vi "HTTP Client Abstract Tree.vi"() -> ()   [LabVIEW 2021]
uses:
  Classes/HTTP Client Base/HTTP Client Base.lvclass
  C:/Users/bjustice/Documents/GitHub/HTTP-Client-Abstract/lv_src/Classes/HTTP Client Abstract/HTTP Client Abstract.lvclass
  Classes/HTTP Client reqwest/HTTP Client reqwest.lvclass
  Classes/HTTP Client Advanced/HTTP Client Advanced.lvclass
  Classes/HTTP Client Abstract/HTTP Client Abstract.lvclass
panel:
  out "Array":string[][](array[string])
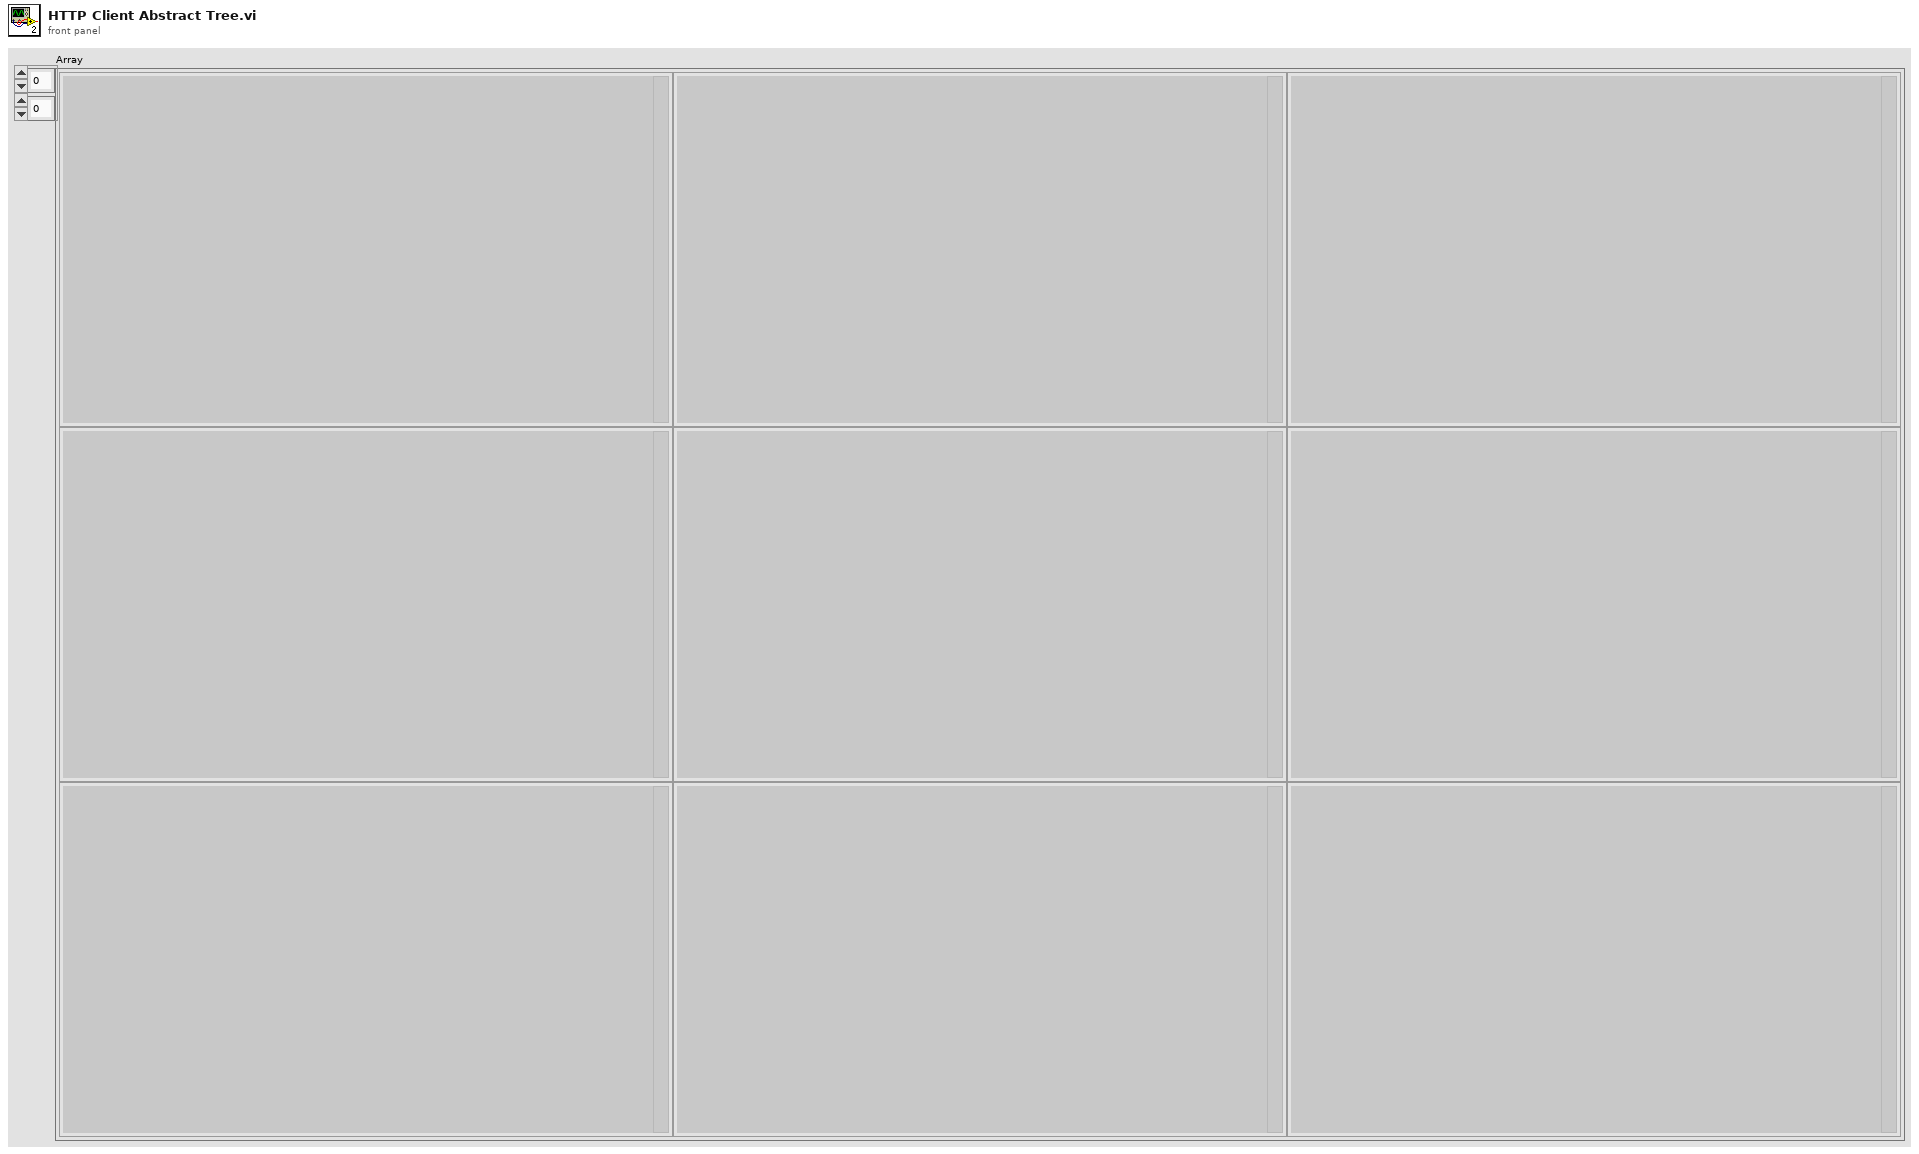
[diagram p1: front panel]
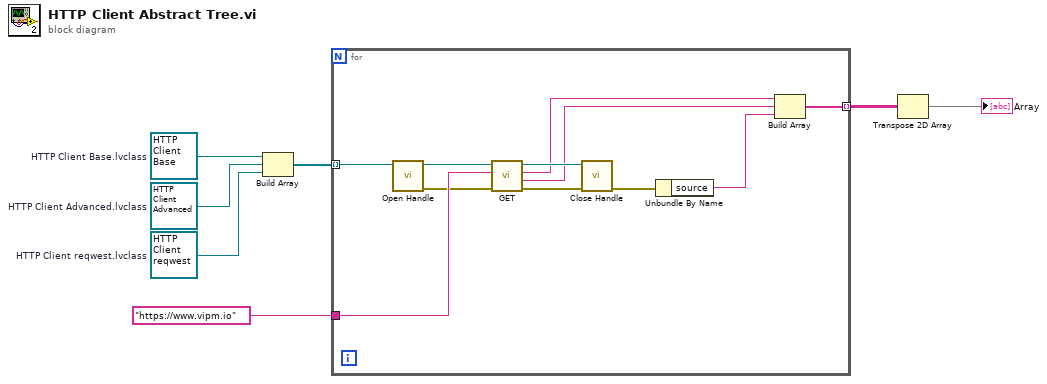
[diagram p0: block diagram]
diagram:
  w7 = refnum<class "HTTP Client Advanced.lvclass"> refnum  # HTTP Client Advanced.lvclass
  w5 = refnum<class "HTTP Client reqwest.lvclass"> refnum  # HTTP Client reqwest.lvclass
  w6 = refnum<class "HTTP Client Base.lvclass"> refnum  # HTTP Client Base.lvclass
  n1 = Build Array(w6, w7, w5) -> (w4:refnum<class "HTTP Client Abstract.lvclass">[])
  n2 = for {
    tunnel: w4 -> [w18] mode=indexing
    tunnel: "https://www.vipm.io" ("url") -> [w15]
    tunnel: [w9] -> w2 mode=indexing
    n3 = call-dynamic "Open Handle.vi"("HTTP Client Abstract in"=w18) -> ("error out"=w14:errorcluster, "HTTP Client Abstract out"=w17:refnum<class "HTTP Client Abstract.lvclass">)  [unwired: 9 in]
    n4 = call-dynamic "GET.vi"("error in (no error)"=w14, "url"=w15, "HTTP Client Abstract in"=w17) -> ("error out"=w13:errorcluster, "body"=w8:string, "headers"=w11:string, "HTTP Client Abstract out"=w16:refnum<class "HTTP Client Abstract.lvclass">)  [unwired: 5 in]
    n5 = call-dynamic "Close Handle.vi"("error in (no error)"=w13, "HTTP Client Abstract in"=w16) -> ("error out"=w12:errorcluster)  [unwired: 8 in, 1 out]
    n6 = Unbundle By Name(w12) -> ("source"=w10:string)
    n7 = Build Array(w11, w8, w10) -> (w9:string[])
  }
  n8 = Transpose 2D Array(2D array=w2) -> (transposed array=→"Array":string[][])
